vi "Stream_data_171213.vi"(7 "VISA resource name in":refnum<visa-resource-name>, 8 "error in (no error)":errorcluster, 9 "Notifier error in":errorcluster, 10 "Play / Pause":bool, 11 "Notifier in":refnum<notifier>) -> (0 "VISA error out":errorcluster, 1 "Notifier error out":errorcluster, 2 "read buffer":string, 3 "VISA Refnum out":refnum<visa-resource-name>)   [LabVIEW 2016]
uses:
  <vilib>/Instr/_visa.llb/VISA Flush IO Buffer Mask.ctl
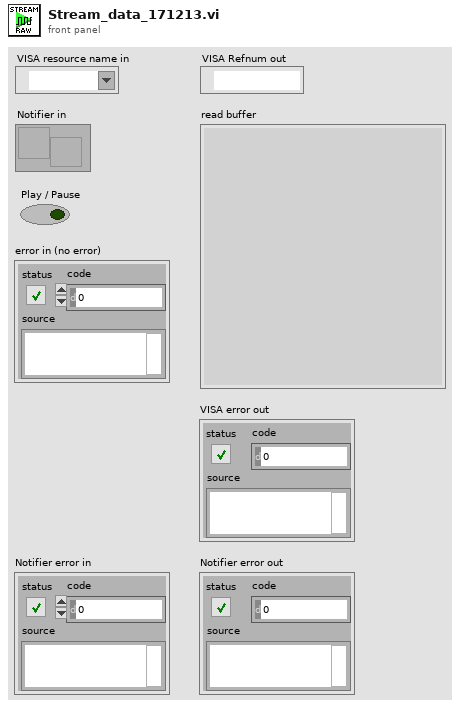
[diagram p1: front panel]
types:
  T1 = typedef "VISA Flush IO Buffer Mask.ctl" = u16
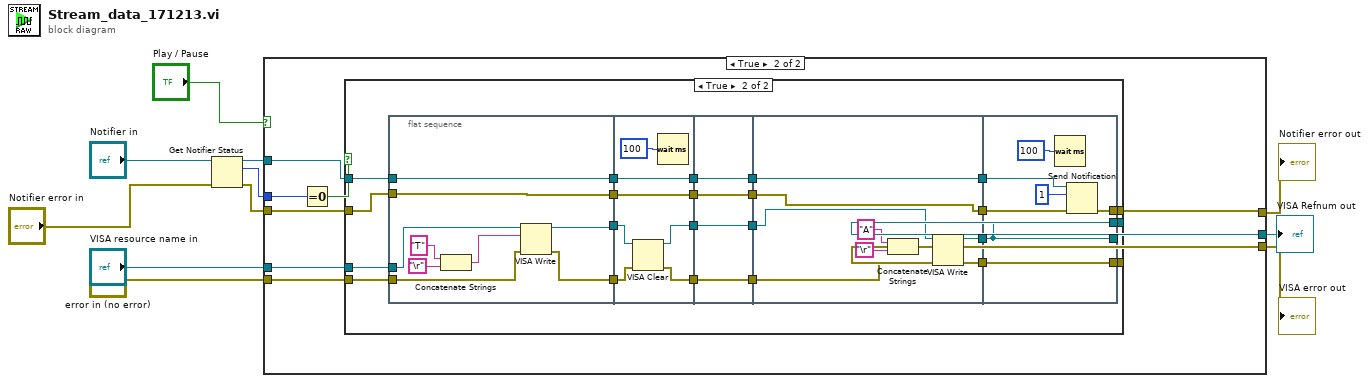
[diagram p0: block diagram]
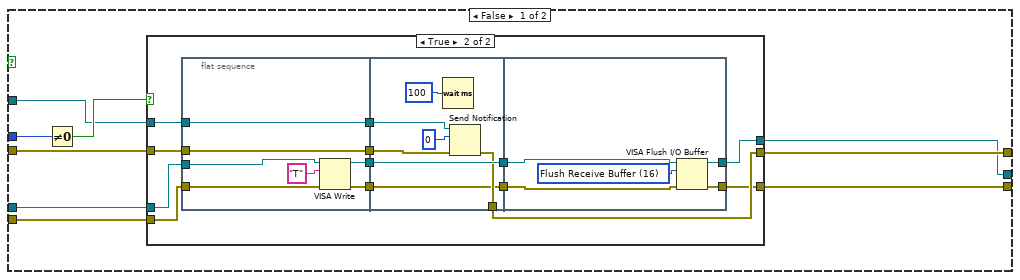
[diagram p2: hidden frame]
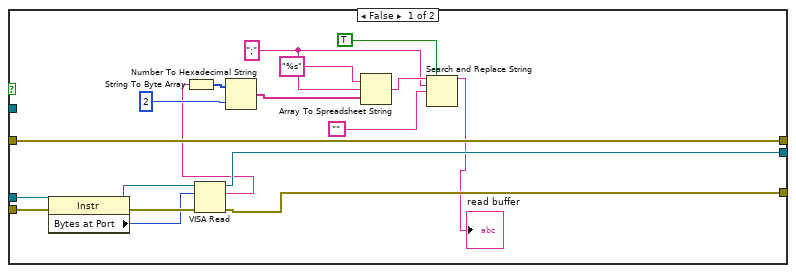
[diagram p4: hidden frame]
diagram:
  n1 = Get Notifier Status(notifier="Notifier in", error in (no error)="Notifier error in") -> (notifier out=w8:refnum<notifier>, current notification=w11:i32, error out=w9:errorcluster)  [unwired: 2 out]
  n2 = case shown="True" "Play / Pause" {
    tunnel: [w12 w56] -> w1
    tunnel: [w13 w57] -> w2
    tunnel: w11 -> [w20 w63]
    tunnel: "error in (no error)" -> [w18 w62]
    tunnel: "VISA resource name in" -> [w17 w61]
    tunnel: w8 -> [w16 w60]
    tunnel: w9 -> [w15 w59]
    tunnel: [w14 w58] -> w10
    frame False {
      n3 = Not Equal To 0?(x=w20) -> (x != 0?=w19:bool)
      n4 = case shown="True" w19 {
        tunnel: w18 -> [w23 w32]
        tunnel: w17 -> [w22 w31]
        tunnel: w16 -> [_ w30]
        tunnel: w15 -> [w21 w29]
        tunnel: [w21 w28] -> w14
        tunnel: [w22 w27] -> w13
        tunnel: [w23 w26] -> w12
        frame False {
        }
        frame True {
          n5 = flat-sequence {
            tunnel: w31 -> [w43]
            tunnel: w32 -> [w42]
            tunnel: [w41] -> w36
            tunnel: [w40] -> w35
            tunnel: [w39] -> w34
            tunnel: w30 -> [w39]
            tunnel: [w38] -> w33
            tunnel: w29 -> [w38]
            tunnel: w36 -> [w49]
            tunnel: w35 -> [w44]
            tunnel: [w48] -> w28
            tunnel: w34 -> [w47]
            tunnel: w33 -> [w46]
            tunnel: [w49] -> w25
            tunnel: [w44] -> w24
            tunnel: [w55] -> w26
            tunnel: [w52] -> w27
            tunnel: w25 -> [w53]
            tunnel: w24 -> [w54]
            frame #0 {
              n6 = VISA Write(VISA resource name=w43, write buffer="T", error in (no error)=w42) -> (VISA resource name out=w41:refnum<visa-resource-name>, error out=w40:errorcluster)  [unwired: 1 out]
            }
            frame #1 {
              n7 = Wait (ms)(milliseconds to wait=u32 100) -> ()  [unwired: 1 out]
              n8 = Send Notification(notification=0, notifier=w47, error in (no error)=w46) -> (error out=w48:errorcluster)  [unwired: 1 out]
            }
            frame #2 {
              w51 = T1 16 items=["Flush Receive Buffer"=16, "Write Transmit Buffer to Device"=32, "Flush Receive Buffer (No I/O)"=64, "Flush Transmit Buffer"=128] ("Mask")
              n9 = VISA Flush I/O Buffer(VISA resource name=w53, mask (16)=w51, error in (no error)=w54) -> (VISA resource name out=w52:refnum<visa-resource-name>, error out=w55:errorcluster)
            }
          }
        }
      }
    }
    frame True {
      n10 = Equal To 0?(x=w63) -> (x = 0?=w64:bool)
      n11 = case shown="True" w64 {
        tunnel: w62 -> [w82 w101]
        tunnel: w61 -> [w81 w100]
        tunnel: w60 -> [_ w99]
        tunnel: w59 -> [w75 w98]
        tunnel: [w75 w97] -> w58
        tunnel: [w77 w96] -> w57
        tunnel: [w76 w95] -> w56
        frame False {
          w69 = ";" ("delimiter (Tab)")
          n12 = property class="Instr"(reference=w81, error in=w82) -> (reference out=w80:refnum<visa-resource-name>, error out=w79:errorcluster, "Bytes at Port"=w78:u32)
          n13 = VISA Read(VISA resource name=w80, byte count=w78, error in (no error)=w79) -> (VISA resource name out=w77:refnum<visa-resource-name>, read buffer=w67:string, error out=w76:errorcluster)  [unwired: 1 out]
          n14 = String To Byte Array(string=w67) -> (unsigned byte array=w74:u8[])
          n15 = Number To Hexadecimal String(1:i16 2 ("width (-)"), 2:w74) -> (0:w72:string[])
          n16 = Array To Spreadsheet String(delimiter (Tab)=w69, array=w72, 3:"%s" ("format string")) -> (spreadsheet string=w70:string)
          n17 = Search and Replace String(replace all?=TRUE ("replace all? (F)"), input string=w70, search string=w69, replace string="") -> (result string=→"read buffer":string)  [unwired: 4 in, 3 out]
        }
        frame True {
          n18 = flat-sequence {
            tunnel: w101 -> [w110]
            tunnel: w100 -> [w111]
            tunnel: w98 -> [w113]
            tunnel: w99 -> [w114]
            tunnel: [w114] -> w94
            tunnel: [w113] -> w93
            tunnel: [w112] -> w92
            tunnel: [w109] -> w91
            tunnel: w94 -> [w121]
            tunnel: [w121] -> w90
            tunnel: w93 -> [w120]
            tunnel: [w120] -> w88
            tunnel: w92 -> [w116]
            tunnel: [w115] -> w86
            tunnel: w91 -> [w118]
            tunnel: [w117] -> w84
            tunnel: w90 -> [w125]
            tunnel: [w125] -> w89
            tunnel: w88 -> [w124]
            tunnel: [w124] -> w87
            tunnel: w86 -> [w123]
            tunnel: [w123] -> w85
            tunnel: w84 -> [w122]
            tunnel: [w122] -> w83
            tunnel: [w131] -> w105
            tunnel: [w130] -> w104
            tunnel: [w127] -> w103
            tunnel: [w126] -> w102
            tunnel: w89 -> [w131]
            tunnel: w87 -> [w130]
            tunnel: w85 -> [w129]
            tunnel: w83 -> [w128]
            tunnel: w105 -> [w140]
            tunnel: w104 -> [w139]
            tunnel: [w137] -> w97
            tunnel: [w136] -> w95
            tunnel: w103 -> [w136]
            tunnel: [w135] -> _
            tunnel: w102 -> [w135]
            tunnel: [w135] -> w96
            frame #0 {
              n19 = Concatenate Strings("T" ("write buffer"), "\r") -> (w106:string)
              n20 = VISA Write(VISA resource name=w111, write buffer=w106, error in (no error)=w110) -> (VISA resource name out=w112:refnum<visa-resource-name>, error out=w109:errorcluster)  [unwired: 1 out]
            }
            frame #1 {
              n21 = VISA Clear(VISA resource name=w116, error in (no error)=w118) -> (VISA resource name out=w115:refnum<visa-resource-name>, error out=w117:errorcluster)
              n22 = Wait (ms)(milliseconds to wait=u32 100) -> ()  [unwired: 1 out]
            }
            frame #2 {
            }
            frame #3 {
              n23 = Concatenate Strings("A" ("write buffer"), "\r") -> (w132:string)
              n24 = VISA Write(VISA resource name=w129, write buffer=w132, error in (no error)=w128) -> (VISA resource name out=w126:refnum<visa-resource-name>, error out=w127:errorcluster)  [unwired: 1 out]
            }
            frame #4 {
              n25 = Wait (ms)(milliseconds to wait=u32 100) -> ()  [unwired: 1 out]
              n26 = Send Notification(notification=1, notifier=w140, error in (no error)=w139) -> (error out=w137:errorcluster)  [unwired: 1 out]
            }
          }
        }
      }
    }
  }
  "Notifier error out" <- w10
  "VISA Refnum out" <- w2
  "VISA error out" <- w1
